vi "Test Broadcast Latest Message Data.vi"(8 "error in (no error)":errorcluster, 11 "Test Case In":refnum<class "Debugger Test.lvclass">) -> (0 "error out":errorcluster, 3 "Test Case Out":refnum<class "Debugger Test.lvclass">)   [LabVIEW 2020, in "Debugger Test.lvclass"]
uses:
  Debugger Test.lvclass
  Debugger Test.lvclass/Debugger Test.ctl
  01074fa8-ee8a-411d-bc8b-fc92c4f90959.vi
  source/Process/Debug Process.lvclass
  source/Debugger/Debugger.lvclass
  source/Debug Data/Debug Data.lvclass
  source/Debug Data/Raw Debug Data.ctl
  C:/Users/anton/Documents/GitHub/triarc-debugger/source/Process/Debug Process.lvclass
  C:/Users/anton/Documents/GitHub/triarc-debugger/source/Debugger/Debugger.lvclass
  C:/Users/anton/Documents/GitHub/triarc-debugger/source/Debug Data Event/Debug Data Listener.lvclass
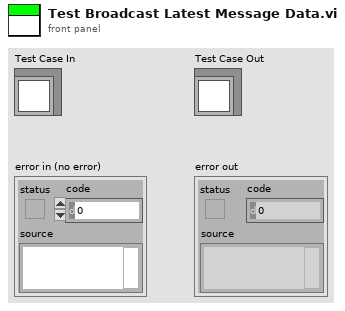
[diagram p1: front panel]
types:
  T1 = typedef "Debug Data.lvclass/Raw Debug Data.ctl" = cluster{"Action":string, "Call Chain":string, "Process":string, "Message":string, "Message Data":variant, "Time":dbl}
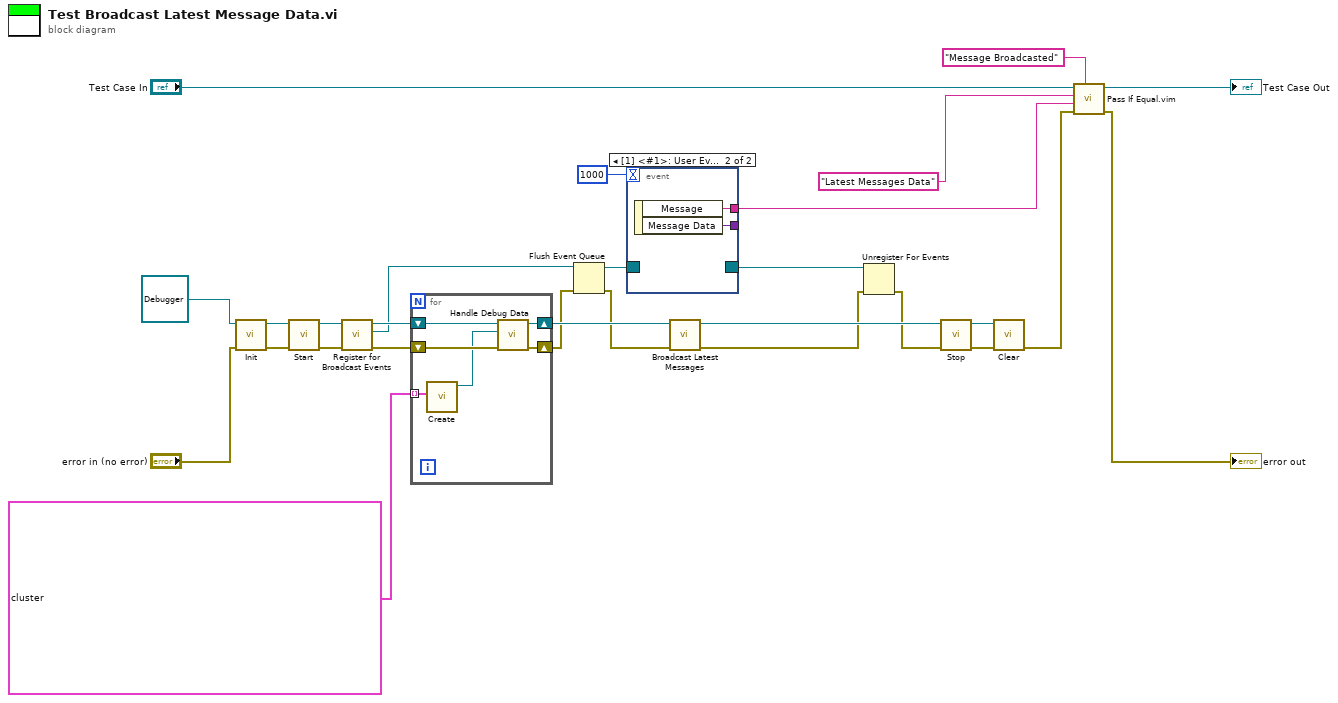
[diagram p0: block diagram]
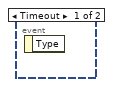
[diagram p2: hidden frame]
diagram:
  n1 = call-dynamic "Init.vi"("error in (no error)"="error in (no error)", "Process In"=refnum<class "Debugger.lvclass"> refnum ("Debug Data Event In 2")) -> ("error out"=w24:errorcluster, "Process Out"=w25:refnum<class "Debugger.lvclass">)  [unwired: 8 in]
  n2 = call "Start.vi"("error in (no error)"=w24, "Process In"=w25) -> ("error out"=w22:errorcluster, "Process Out"=w23:refnum<class "Debugger.lvclass">)  [unwired: 7 in, 1 out]
  n3 = call "Register for Broadcast Events.vi"("error in (no error)"=w22, "Process In"=w23) -> ("error out"=w21:errorcluster, "Event Registration Refnum Out"=w7:refnum<event-registration>, "Process Out"=w15:refnum<class "Debugger.lvclass">)  [unwired: 7 in]
  n4 = for {
    shift-right: [w32] -> w19
    shift-left: w21 -> [w34]
    shift-right: [w33] -> w20
    shift-left: w15 -> [w31]
    tunnel: T1[] [{"Action"="Send", "Call Chain"="Test.vi:123456", "Process"="Process 1", "Message"="Init", "Message Data"=variant, "Time"=0.0}, {"Action"="Receive", "Call Chain"="TF.lvlib:Process.lvclass:Handle Messages.vi:1960001", "Process"="Process 1", "Message"="Init", "Message Data"=variant, "Time"=0.0}, {"Action"="Send", "Call Chain"="Test.vi", "Process"="Process 1", "Message"="Start", "Message Data"=variant, "Time"=0.0}] ("Debug Data Cluster") -> [w29] mode=indexing
    n5 = call "Create.vi"("Debug Data Cluster"=w29) -> ("Debug Data out"=w30:refnum<class "Debug Data.lvclass">)  [unwired: 9 in, 1 out]
    n6 = call-dynamic "Handle Debug Data.vi"("error in (no error)"=w34, "Debug Data.lvclass"=w30, "Debug Data Event In"=w31) -> ("error out"=w32:errorcluster, "Debug Data Event Out"=w33:refnum<class "Debugger.lvclass">)  [unwired: 7 in]
  }
  n7 = Flush Event Queue(0:w7, 3:w19) -> (8:w6:refnum<event-registration>, 11:w8:errorcluster)  [unwired: 4 in, 1 out]
  n8 = event shown="[1] <#1>: User Event" {
    selector: w6 -> [_ _]
    dyn-events: [_ _] -> w10
    timeout: 1000 -> [_ _]
    tunnel: [_ w36] -> _
    tunnel: [_ w35] -> w2
    event Timeout {
      n9 = event-data() -> ()  [unwired: 1 in, 1 out]
    }
    event User Event {
      n10 = event-data() -> ("Message"=w35:string, "Message Data"=w36:variant)  [unwired: 1 in]
    }
  }
  n11 = call "Broadcast Latest Messages.vi"("error in (no error)"=w8, "Debugger in"=w20) -> ("error out"=w5:errorcluster, "Debugger out"=w18:refnum<class "Debugger.lvclass">)  [unwired: 8 in]
  n12 = Unregister For Events(event registration refnum=w10, error in=w5) -> (error out=w4:errorcluster)
  n13 = call "Stop.vi"("error in (no error)"=w4, "Process In"=w18) -> ("error out"=w16:errorcluster, "Process Out"=w17:refnum<class "Debugger.lvclass">)  [unwired: 7 in, 1 out]
  n14 = call-dynamic "Clear.vi"("error in (no error)"=w16, "Process In"=w17) -> ("error out"=w12:errorcluster)  [unwired: 9 in]
  n15 = call "Pass If Equal.vim"("Description"="Message Broadcasted", "error in (no error)"=w12, "Actual"=w2, "Expected"="Latest Messages Data" ("Message"), "LUnit Test Case In"="Test Case In") -> ("error out"=→"error out":errorcluster, "LUnit Test Case Out"=→"Test Case Out":refnum<class "Debugger Test.lvclass">)  [unwired: 5 in]
